vi "Close.vi"(8 "error in (no error)":errorcluster, 11 "Subpanel.lvclass":refnum<class "Subpanel.lvclass">) -> (0 "error out":errorcluster, 3 "Subpanel out":refnum<class "Subpanel.lvclass">)   [LabVIEW 2019, in "Subpanel.lvclass"]
uses:
  Subpanel.lvclass
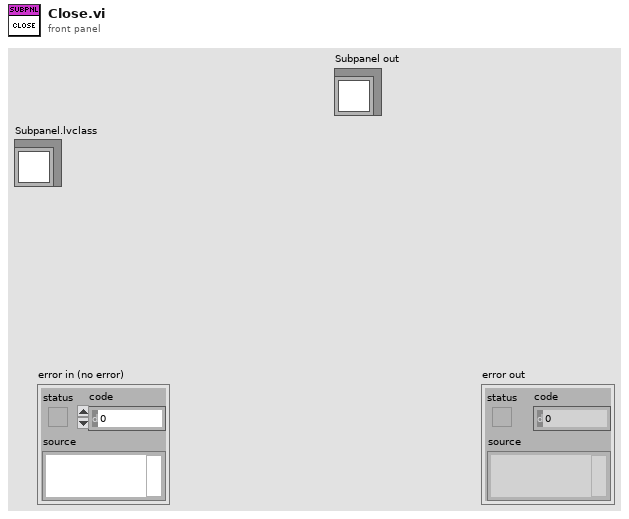
[diagram p1: front panel]
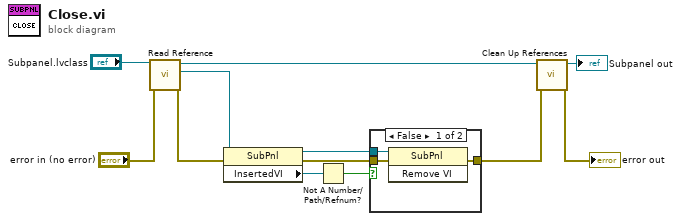
[diagram p0: block diagram]
diagram:
  n1 = call-dynamic "Read Reference.vi"("error in (no error)"="error in (no error)", "Subpanel in"="Subpanel.lvclass") -> ("error out"=w3:errorcluster, "Reference"=w5:refnum<vi>, "Subpanel out"=w2:refnum<class "Subpanel.lvclass">)  [unwired: 7 in]
  n2 = property class="SubPnl"(reference=w5, error in=w3) -> (reference out=w12:refnum<vi>, error out=w9:errorcluster, "InsertedVI"=w10:refnum<vi>)
  n3 = Not A Number/Path/Refnum?(number/path/refnum=w10) -> (NaN/Path/Refnum?=w11:bool)
  n4 = case shown="False" w11 {
    tunnel: w12 -> [w15 _]
    tunnel: w9 -> [w14 w16]
    tunnel: [w13 w16] -> w7
    frame False {
      n5 = invoke class="SubPnl" method="Remove VI"(reference=w15, error in=w14) -> (error out=w13:errorcluster)  [unwired: 1 in, 2 out]
    }
    frame True {
    }
  }
  n6 = call-dynamic "Clean Up References.vi"("error in (no error)"=w7, "Subpanel in"=w2) -> ("error out"=→"error out":errorcluster, "Subpanel out"=→"Subpanel out":refnum<class "Subpanel.lvclass">)  [unwired: 8 in]
